vi "HFRR ADV v024 new software.vi"() -> ()   [LabVIEW 2025] (continued)
                  n3489 = property on="Air Temperature  ( °C )" class="XYGraph (strict)"("Y Scale.Name Label.Text"=w4683) -> ()  [unwired: 2 in, 2 out]
                }
                frame 82 {
                  n3490 = local write "S 84"(w4684) -> ()
                }
                frame 83 {
                  n3491 = local write "S 85"(w4685) -> ()
                }
                frame 84 {
                  n3492 = local write "S 86"(w4686) -> ()
                }
                frame 85 {
                  n3493 = local write "S 87"(w4687) -> ()
                }
                frame 86 {
                  n3494 = local write "S 88"(w4688) -> ()
                }
                frame 87 {
                }
                frame 88 {
                  n3495 = local write "S 90"(w4690) -> ()
                }
                frame 89 {
                  n3496 = local write "S 91"(w4691) -> ()
                }
                frame 90 {
                  n3497 = local write "S 92"(w4692) -> ()
                }
                frame 91 {
                  n3498 = local write "S 93"(w4693) -> ()
                }
                frame 92 {
                  n3499 = local write "S 94"(w4694) -> ()
                }
                frame 93 {
                  n3500 = local write "S 95"(w4695) -> ()
                }
                frame 94 {
                  n3501 = local write "S 96"(w4696) -> ()
                }
                frame 95 {
                  n3502 = local write "S 97"(w4697) -> ()
                }
                frame 96 {
                  n3503 = local write "S 98"(w4698) -> ()
                }
                frame 97 {
                  n3504 = local write "S 99"(w4699) -> ()
                }
                frame 98 {
                  n3505 = local write "S 100"(w4700) -> ()
                }
                frame 99 {
                  n3506 = local write "S 101"(w4701) -> ()
                }
                frame 100 {
                  n3507 = local write "S 102"(w4702) -> ()
                }
                frame 101 {
                  n3508 = local write "S 103"(w4703) -> ()
                }
                frame 102 {
                  n3509 = local write "S 104"(w4704) -> ()
                }
                frame 103 {
                  n3510 = local write "S 105"(w4705) -> ()
                }
                frame 104 {
                  n3511 = local write "S 106"(w4706) -> ()
                }
                frame 105 {
                }
                frame 106 {
                  n3512 = property on="OK Button 17" class="Bool (strict)"("Boolean Text.Text"=w4707) -> ()  [unwired: 2 in, 2 out]
                }
                frame 107 {
                  n3513 = property on="OK Button 16" class="Bool (strict)"("Boolean Text.Text"=w4708) -> ()  [unwired: 2 in, 2 out]
                }
                frame 108 {
                  n3514 = property on="TITTLE" class="Str"("Caption.Text"=w4709) -> ()  [unwired: 2 in, 2 out]
                }
                frame 109 {
                  "String 30" <- w4710
                }
                frame 110 {
                  n3515 = property on="Test Date" class="Str"("Caption.Text"=w4711) -> ()  [unwired: 2 in, 2 out]
                  "String 31" <- w4711
                }
                frame 111 {
                  n3516 = property on="Sample ID" class="Str"("Caption.Text"=w4712) -> ()  [unwired: 2 in, 2 out]
                  "String 32" <- w4712
                }
                frame 112 {
                  n3517 = property on="Tested by" class="Str"("Caption.Text"=w4713) -> ()  [unwired: 2 in, 2 out]
                  "String 33" <- w4713
                }
                frame 113 {
                  n3518 = property on="System Configured Printers 2" class="Arr (strict)"("Caption.Text"=w4714) -> ()  [unwired: 2 in, 2 out]
                }
                frame 114 {
                  n3519 = property on="Selected Printer" class="Str"("Caption.Text"=w4715) -> ()  [unwired: 2 in, 2 out]
                }
                frame 115 {
                  n3520 = property on="Select Printer 3" class="DigNum (strict)"("Caption.Text"=w4716) -> ()  [unwired: 2 in, 2 out]
                }
                frame 116 {
                  n3521 = property on="Print" class="Bool (strict)"("Boolean Text.Text"=w4717) -> ()  [unwired: 2 in, 2 out]
                }
                frame 117 {
                  "String 41" <- w4718
                }
                frame 118 {
                  n3522 = property on="tested by" class="Str"("Caption.Text"=w4719) -> ()  [unwired: 2 in, 2 out]
                }
                frame 119 {
                }
                frame 120 {
                  n3523 = property on="Export" class="Bool (strict)"("Boolean Text.Text"=w4720) -> ()  [unwired: 2 in, 2 out]
                }
                frame 121 {
                  n3524 = property on="TEMP INTERCEPT:" class="DigNum (strict)"("Caption.Text"=w4721) -> ()  [unwired: 2 in, 2 out]
                }
                frame 122 {
                  n3525 = property on="AIR TEMP INTERCEPT:" class="DigNum (strict)"("Caption.Text"=w4722) -> ()  [unwired: 2 in, 2 out]
                }
                frame 123 {
                  n3526 = property on="Select File Type" class="Enum (strict)"("Caption.Text"=w4723) -> ()  [unwired: 2 in, 2 out]
                }
                frame 124 {
                  n3527 = property on="s.NO" class="Str"("Caption.Text"=w4724) -> ()  [unwired: 2 in, 2 out]
                  "String 45" <- w4724
                }
                frame 125 {
                  n3528 = property on="trip1 8" class="Bool (strict)"("Boolean Text.Text"=w4725) -> ()  [unwired: 2 in, 2 out]
                }
                frame 126, Default {
                }
              }
            }
          }
          frame #1 {
            w4733 = TRUE ("Visible")
            n3529 = local read "S 91"() -> (w4750:string)
            n3530 = local read "S 90"() -> (w4749:string)
            n3531 = local read "S 88"() -> (w4748:string)
            n3532 = property on="File Path" class="Path"("Caption.Text"=w4749) -> ()  [unwired: 2 in, 2 out]
            n3533 = property on="SrvM CP" class="Bool (strict)"("Boolean Text.Text"=w4748) -> ()  [unwired: 2 in, 2 out]
            n3534 = local read "S 71"() -> (w4743:string)
            n3535 = local read "S 86"() -> (w4745:string)
            n3536 = local read "S 85"() -> (w4746:string)
            n3537 = local read "S 87"() -> (w4744:string)
            n3538 = local read "S 84"() -> (w4747:string)
            n3539 = local read "S 103"() -> (w4732:string)
            n3540 = local read "S 104"() -> (w4731:string)
            n3541 = property on="ENTER THE NEW PASSWORD" class="Str"("Caption.Text"=w4744) -> ()  [unwired: 2 in, 2 out]
            n3542 = property on="Password" class="Str"("Caption.Text"=w4746) -> ()  [unwired: 2 in, 2 out]
            n3543 = property on="ENTER CURRENT PASSWORD" class="Str"("Caption.Text"=w4745) -> ()  [unwired: 2 in, 2 out]
            n3544 = property on="EDIT" class="Bool (strict)"("Boolean Text.Text"=w4743) -> ()  [unwired: 2 in, 2 out]
            n3545 = property on="SAVE" class="Bool (strict)"("Boolean Text.Text"=w4747) -> ()  [unwired: 2 in, 2 out]
            n3546 = Build Array(w4732, w4731) -> (w4730:string[])
            n3547 = property on="Heater Button" class="Bool (strict)"("Strings [4]"=w4730) -> ()  [unwired: 2 in, 2 out]
            n3548 = local read "S 92"() -> (w4742:string)
            n3549 = local read "S 93"() -> (w4741:string)
            n3550 = local read "S 105"() -> (w4728:string)
            n3551 = local read "S 106"() -> (w4727:string)
            n3552 = Build Array(w4742, w4741) -> ()  [unwired: 1 out]
            n3553 = Build Array(w4728, w4727) -> (w4729:string[])
            n3554 = local read "S 95"() -> (w4739:string)
            n3555 = local read "S 94"() -> (w4740:string)
            n3556 = local read "bs"() -> (w4755:string)
            n3557 = local read "as"() -> (w4756:string)
            n3558 = property on="Humidity" class="Bool (strict)"("Strings [4]"=w4729) -> ()  [unwired: 2 in, 2 out]
            n3559 = Concatenate Strings(w4755, "\r", w4756) -> ()  [unwired: 1 out]
            n3560 = property on="STROKE GAIN :" class="DigNum (strict)"("Caption.Text"=w4739) -> ()  [unwired: 2 in, 2 out]
            n3561 = property on="DISPLACEMENT :" class="DigNum (strict)"("Caption.Text"=w4740) -> ()  [unwired: 2 in, 2 out]
            n3562 = property on="Rh After" class="DigNum (strict)"("Caption.Size to Text?"=TRUE ("Caption.Size to Text")) -> ()  [unwired: 2 in, 2 out]
            n3563 = local read "S 48"() -> (w4779:string)
            n3564 = local read "S 50"() -> (w4777:string)
            n3565 = local read "S 51"() -> (w4776:string)
            n3566 = local read "S 49"() -> (w4778:string)
            n3567 = local read "S 52"() -> (w4775:string)
            n3568 = local read "as"() -> (w4760:string)
            n3569 = local read "bs"() -> (w4761:string)
            n3570 = local read "S 56"() -> (w4774:string)
            n3571 = local read "S 57"() -> (w4773:string)
            n3572 = local read "S 58"() -> (w4772:string)
            n3573 = local read "S 59"() -> (w4771:string)
            n3574 = property on="OPEN" class="Bool (strict)"("Boolean Text.Text"=w4775) -> ()  [unwired: 2 in, 2 out]
            n3575 = property on="OPEN 1" class="Bool (strict)"("Boolean Text.Text"=w4779) -> ()  [unwired: 2 in, 2 out]
            n3576 = property on="OPEN 2" class="Bool (strict)"("Boolean Text.Text"=w4778) -> ()  [unwired: 2 in, 2 out]
            n3577 = property on="OPEN 3" class="Bool (strict)"("Boolean Text.Text"=w4777) -> ()  [unwired: 2 in, 2 out]
            n3578 = property on="OPEN 4" class="Bool (strict)"("Boolean Text.Text"=w4776) -> ()  [unwired: 2 in, 2 out]
            n3579 = Concatenate Strings(w4761, "\r", w4760) -> ()  [unwired: 1 out]
            n3580 = local read "S 102"() -> (w4734:string)
            n3581 = property on="КОФ1" class="DigNum (strict)"("Caption.Text"=w4774) -> ()  [unwired: 2 in, 2 out]
            n3582 = local read "S 98"() -> (w4738:string)
            n3583 = local read "S 99"() -> (w4737:string)
            n3584 = local read "S 100"() -> (w4736:string)
            n3585 = local read "S 101"() -> (w4735:string)
            n3586 = property on="КОФ2" class="DigNum (strict)"("Caption.Text"=w4773) -> ()  [unwired: 2 in, 2 out]
            n3587 = property on="КОФ3" class="DigNum (strict)"("Caption.Text"=w4772) -> ()  [unwired: 2 in, 2 out]
            n3588 = property on="КОФ4" class="DigNum (strict)"("Caption.Text"=w4771) -> ()  [unwired: 2 in, 2 out]
            n3589 = local read "bs"() -> (w4759:string)
            n3590 = local read "as"() -> (w4758:string)
            n3591 = local read "S 60"() -> (w4770:string)
            n3592 = local read "S 54"() -> (w4780:string)
            n3593 = Concatenate Strings(w4759, "\r", w4758) -> ()  [unwired: 1 out]
            n3594 = Concatenate Strings(w4780, w4770) -> ()  [unwired: 1 out]
            n3595 = local read "S 77"() -> (→"String 43":string)
            n3596 = local read "S 76"() -> (w4753:string)
            n3597 = local read "S 78"() -> (w4752:string)
            n3598 = local read "S 71"() -> (w4764:string)
            n3599 = local read "S 66"() -> (w4769:string)
            n3600 = local read "S 67"() -> (w4768:string)
            n3601 = local read "S 68"() -> (w4767:string)
            n3602 = local read "S 69"() -> (w4766:string)
            n3603 = local read "S 70"() -> (w4765:string)
            n3604 = property on="AIR TEMP" class="DigNum (strict)"("Caption.Text"=w4752) -> ()  [unwired: 2 in, 2 out]
            n3605 = property on="Set Strk" class="DigNum (strict)"("Caption.Text"=w4753) -> ()  [unwired: 2 in, 2 out]
            n3606 = property on="FRIC. FORCE :" class="DigNum (strict)"("Caption.Text"=w4769) -> ()  [unwired: 2 in, 2 out]
            n3607 = property on="TEMPERATURE :" class="DigNum (strict)"("Caption.Text"=w4768) -> ()  [unwired: 2 in, 2 out]
            n3608 = property on="SPEED OUT:" class="DigNum (strict)"("Caption.Text"=w4767) -> ()  [unwired: 2 in, 2 out]
            n3609 = property on="AIR TEMPERATURE :" class="DigNum (strict)"("Caption.Text"=w4766) -> ()  [unwired: 2 in, 2 out]
            n3610 = property on="HUMIDITY:" class="DigNum (strict)"("Caption.Text"=w4765) -> ()  [unwired: 2 in, 2 out]
            n3611 = property on="EDIT" class="Bool (strict)"("Boolean Text.Text"=w4764) -> ()  [unwired: 2 in, 2 out]
            n3612 = local read "S 79"() -> (w4751:string)
          }
          frame #2 {
          }
        }
        n3613 = local write "Lan flag"(10.0 ("Lan flag")) -> ()
      }
      frame Enabled {
      }
    }
    n3614 = Wait (ms)(milliseconds to wait=u32 2000) -> ()  [unwired: 1 out]
    n3615 = local read "Quit"() -> (w4554:bool)
  }
  n3616 = while {
    shift-right: [w4786] -> _
    shift-left: _ -> [w4787]
    shift-right: [w4784] -> _
    shift-left: T18 {"Read Heave and Surge"="", "Bytes at Heave Port"=0.0, "Heave and Surge COM Port:"="COM9", "Com Port 2"="COM7", "Residual Due"="", "Heave COM Status 2"=TRUE, "Heave COM Status"=TRUE, "Port 2"=TRUE, "Sway PPR"=6400.0, "Surge PPR"=6400.0, "Heave PPR"=6400.0, "Sway Pitch"=2.0, "Surge Pitch"=3.0, "Heave Pitch"=4.0, "Sway Pulses/mm"=320.0, "Surge Pulses/mm"=1600.0, "Heave Pulses/mm"=1600.0, "inner loop"=0.0, "Read Heave and Surge 2"="", "String 36"="", "Write S"=FALSE, "WriteCC1"=[""], "Heave COM Loop"=0, "LastCom"="", "EXIT"=FALSE, "Error Heave"={"status"=TRUE, "code"=-1073807343, "source"=""}} -> [w4783]
    shift-right: [w4781] -> _
    shift-left: enum16{"init", "MAIN", "Panel Close"}."init" -> [w4782]
    stop <- w4785 stop-if-true
    # "HUMIDITY LOOP LOGIC"
    n3617 = case shown="\"MAIN\"" w4782 {
      tunnel: w4787 -> [w4801 w4818 w4875 w4877]
      tunnel: [w4796 w4823 w4875 w4877] -> w4786
      tunnel: [_ _ TRUE _] -> w4785
      tunnel: [w4793 w4821 w4873 w4876] -> w4784
      tunnel: w4783 -> [w4798 w4817 w4873 w4876]
      tunnel: [enum16{"init", "MAIN", "Panel Close"}."MAIN" w4812 _ _] -> w4781
      frame "init" {
        n3618 = local read "Com Port 1"() -> (w4790:refnum<visa-resource-name>)
        n3619 = Bundle By Name(cluster=w4798, "Heave and Surge COM Port:"=w4790) -> (w4797:T18)
        n3620 = call "Instrument fgv uno.vi"("Enum"=T31."INIT", "error in (no error) 2"=w4801, "INPUT"=w4797) -> ("error"=w4799:errorcluster, "output"=w4795:T18)  [unwired: 6 in, 1 out]
        n3621 = case shown="Error" w4799 {
          selector: w4799 -> [w4803 _]
          tunnel: [w4803 w4807] -> w4796
          tunnel: w4795 -> [w4802 w4805]
          tunnel: [w4802 w4804] -> w4794
          frame No Error {
          }
          frame Error {
            n3622 = call "Instrument fgv uno.vi"("Enum"=T31."ERROR INIT", "INPUT"=w4805) -> ("error"=w4808:errorcluster, "output"=w4804:T18)  [unwired: 7 in, 1 out]
            n3623 = call <vilib>:"Clear Errors.vi"("error in (no error)"=w4808) -> ("error out"=w4807:errorcluster)  [unwired: 5 in, 1 out]
          }
        }
        n3624 = local read "LastCom Humidity"() -> (w4789:string)
        n3625 = Unbundle By Name(w4794) -> ("Heave COM Status 2"=→"COM Status":bool, "Error Heave"=→"Error  2":errorcluster)  [unwired: 1 out]
        n3626 = Bundle By Name(cluster=w4794, "LastCom"=w4789) -> (w4793:T18)
      }
      frame "MAIN" {
        n3627 = Unbundle By Name(w4817) -> ("Com Port 2"=w4825:refnum<visa-resource-name>)
        n3628 = local read "Com Port 1"() -> (w4811:refnum<visa-resource-name>)
        n3629 = local write "Com Port 5"(w4825) -> ()
        n3630 = Bundle By Name(cluster=w4817, "Heave and Surge COM Port:"=w4811) -> (w4816:T18)
        n3631 = Equal?(x=w4825, y=w4811) -> (x = y?=w4824:bool)
        n3632 = case shown="True" w4824 {
          tunnel: [w4829 w4846] -> w4823
          tunnel: w4818 -> [w4830 w4852]
          tunnel: w4816 -> [w4828 w4850]
          tunnel: [w4827 w4845] -> w4821
          frame False {
            n3633 = call <vilib>:"Clear Errors.vi"("error in (no error)"=w4830) -> ("error out"=w4826:errorcluster)  [unwired: 5 in, 1 out]
            n3634 = call "Instrument fgv uno.vi"("Enum"=T31."ERROR INIT", "error in (no error) 2"=w4826, "INPUT"=w4828) -> ("error"=w4832:errorcluster, "output"=w4827:T18)  [unwired: 6 in, 1 out]
            n3635 = call <vilib>:"Clear Errors.vi"("error in (no error)"=w4832) -> ("error out"=w4829:errorcluster)  [unwired: 5 in, 1 out]
          }
          frame True {
            n3636 = call "Instrument fgv uno.vi"("Enum"=T31."READ", "error in (no error) 2"=w4852, "INPUT"=w4850) -> ("error"=w4851:errorcluster, "output"=w4843:T18)  [unwired: 6 in, 1 out]
            n3637 = Bundle By Name(cluster=w4843, "String 36"="WRITE HUMIDITY") -> (w4842:T18)
            n3638 = case shown="True" "Write" {
              selector: "Write" -> [_ w4872]
              tunnel: w4851 -> [w4865 w4871]
              tunnel: [w4865 w4870] -> w4840
              tunnel: w4842 -> [w4864 w4867]
              tunnel: [w4864 w4866] -> w4839
              frame False {
              }
              frame True {
                n3639 = Not(x=w4872) -> (.not. x?=w4868:bool)
                n3640 = local write "Write"(w4868) -> ()
                n3641 = call "Instrument fgv uno.vi"("Enum"=T31."MANUAL WRITE", "error in (no error) 2"=w4871, "INPUT"=w4867) -> ("error"=w4870:errorcluster, "output"=w4866:T18)  [unwired: 6 in, 1 out]
              }
            }
            n3642 = Array Size(array="WriteHumidity") -> (size(s)=w4837:i32)
            n3643 = Greater Than 0?(x=w4837) -> (x > 0?=w4836:bool)
            n3644 = call "Instrument fgv uno.vi"("Enum"=T31."WRITE", "error in (no error) 2"=w4840, "WriteCC1"="WriteHumidity", "INPUT"=w4839) -> ("error"=w4848:errorcluster, "WriteCC1 2"=w4838:string[], "output"=w4847:T18)  [unwired: 5 in]
            n3645 = case shown="True" w4836 {
              tunnel: w4838 -> [_ w4854]
              frame False {
              }
              frame True {
                n3646 = local write "WriteHumidity"(w4854) -> ()
              }
            }
            n3647 = case shown="No Error" w4848 {
              selector: w4848 -> [w4855 w4858]
              tunnel: w4847 -> [w4856 w4863]
              tunnel: [w4856 w4862] -> w4845
              tunnel: [w4855 w4860] -> w4846
              frame No Error {
              }
              frame Error {
                n3648 = call <vilib>:"Clear Errors.vi"("error in (no error)"=w4858) -> ("error out"=w4857:errorcluster)  [unwired: 5 in, 1 out]
                n3649 = call "Instrument fgv uno.vi"("Enum"=T31."ERROR INIT", "error in (no error) 2"=w4857, "INPUT"=w4863) -> ("error"=w4861:errorcluster, "output"=w4862:T18)  [unwired: 6 in, 1 out]
                n3650 = call <vilib>:"Clear Errors.vi"("error in (no error)"=w4861) -> ("error out"=w4860:errorcluster)  [unwired: 5 in, 1 out]
              }
            }
            n3651 = Unbundle By Name(w4845) -> ("LastCom"=→"LastCom Humidity":string, "Read Heave and Surge"=→"Read HUMIDITY":string)
          }
        }
        n3652 = Unbundle By Name(w4821) -> ("Heave COM Status 2"=w4822:bool, "Error Heave"=w4819:errorcluster, "Bytes at Heave Port"=→"Bytes at Humidity Port  2":dbl)  [unwired: 1 out]
        n3653 = Unbundle By Name(w4819) -> ("status"=→"Humidity Port":bool)
        n3654 = Not(x=w4822) -> (.not. x?=w4809:bool)
        n3655 = local read "Quit"() -> (w4813:bool)
        n3656 = local write "COM Status"(w4809) -> ()
        n3657 = Select(t=enum16{"init", "MAIN", "Panel Close"}."Panel Close", s=w4813, f=enum16{"init", "MAIN", "Panel Close"}."MAIN") -> (s? t:f=w4812:enum16{"init", "MAIN", "Panel Close"})
      }
      frame "Panel Close" {
      }
      frame Default {
      }
    }
  }
  n3658 = disable-structure shown="Disabled" {
    frame Disabled {
      n3659 = while {
        tunnel: [w4879] -> _
        i -> [w4879]
        stop <- w4878 continue-if-true
        n3660 = Wait (ms)(milliseconds to wait=u32 50) -> ()  [unwired: 1 out]
        n3661 = stacked-sequence {
          frame #0 {
            # "Controls Text color"
            # "Controls BG color"
            n3662 = property on="FILE" class="Str"("Text.Text Colors:Text Color"="SC  Text") -> ()  [unwired: 2 in, 2 out]
            n3663 = property on="Fuel Discription :" class="Str"("Text.Text Colors:Text Color"="SC  Text") -> ()  [unwired: 2 in, 2 out]
            n3664 = property on="tested by" class="Str"("Text.Text Colors:Text Color"="SC  Text") -> ()  [unwired: 2 in, 2 out]
            n3665 = property on="Remarks :" class="Str"("Text.Text Colors:Text Color"="SC  Text") -> ()  [unwired: 2 in, 2 out]
            n3666 = property class="DigNum (strict)"("Numeric Text.Text Colors:BG Color"="NC BG") -> ()  [unwired: 2 in, 2 out]
            n3667 = property class="DigNum (strict)"("Numeric Text.Text Colors:BG Color"="NC BG") -> ()  [unwired: 2 in, 2 out]
            n3668 = property class="DigNum (strict)"("Numeric Text.Text Colors:BG Color"="NC BG") -> ()  [unwired: 2 in, 2 out]
            n3669 = property class="DigNum (strict)"("Numeric Text.Text Colors:BG Color"="NC BG") -> ()  [unwired: 2 in, 2 out]
            n3670 = property class="DigNum (strict)"("Numeric Text.Text Colors:BG Color"="NC BG") -> ()  [unwired: 2 in, 2 out]
            n3671 = property class="DigNum (strict)"("Numeric Text.Text Colors:BG Color"="NC BG") -> ()  [unwired: 2 in, 2 out]
            n3672 = property class="DigNum (strict)"("Numeric Text.Text Colors:BG Color"="NC BG") -> ()  [unwired: 2 in, 2 out]
            n3673 = property class="DigNum (strict)"("Numeric Text.Text Colors:BG Color"="NC BG") -> ()  [unwired: 2 in, 2 out]
            n3674 = property class="DigNum (strict)"("Numeric Text.Text Colors:BG Color"="NC BG") -> ()  [unwired: 2 in, 2 out]
            n3675 = property class="DigNum (strict)"("Numeric Text.Text Colors:BG Color"="NC BG") -> ()  [unwired: 2 in, 2 out]
            n3676 = property class="DigNum (strict)"("Numeric Text.Text Colors:BG Color"="NC BG") -> ()  [unwired: 2 in, 2 out]
            n3677 = property class="DigNum (strict)"("Numeric Text.Text Colors:BG Color"="NC BG") -> ()  [unwired: 2 in, 2 out]
            n3678 = property on="FILE" class="Str"("Text.Text Colors:BG Color"="SC BG 3") -> ()  [unwired: 2 in, 2 out]
            n3679 = property on="Fuel Discription :" class="Str"("Text.Text Colors:BG Color"="SC BG 3") -> ()  [unwired: 2 in, 2 out]
            n3680 = property on="tested by" class="Str"("Text.Text Colors:BG Color"="SC BG 3") -> ()  [unwired: 2 in, 2 out]
            n3681 = property on="Remarks :" class="Str"("Text.Text Colors:BG Color"="SC BG 3") -> ()  [unwired: 2 in, 2 out]
            n3682 = property class="DigNum (strict)"("Numeric Text.Text Colors:Text Color"="NC Text") -> ()  [unwired: 2 in, 2 out]
            n3683 = property class="DigNum (strict)"("Numeric Text.Text Colors:Text Color"="NC Text") -> ()  [unwired: 2 in, 2 out]
            n3684 = property class="DigNum (strict)"("Numeric Text.Text Colors:Text Color"="NC Text") -> ()  [unwired: 2 in, 2 out]
            n3685 = property class="DigNum (strict)"("Numeric Text.Text Colors:Text Color"="NC Text") -> ()  [unwired: 2 in, 2 out]
            n3686 = property class="DigNum (strict)"("Numeric Text.Text Colors:Text Color"="NC Text") -> ()  [unwired: 2 in, 2 out]
            n3687 = property class="DigNum (strict)"("Numeric Text.Text Colors:Text Color"="NC Text") -> ()  [unwired: 2 in, 2 out]
            n3688 = property class="DigNum (strict)"("Numeric Text.Text Colors:Text Color"="NC Text") -> ()  [unwired: 2 in, 2 out]
            n3689 = property class="DigNum (strict)"("Numeric Text.Text Colors:Text Color"="NC Text") -> ()  [unwired: 2 in, 2 out]
            n3690 = property class="DigNum (strict)"("Numeric Text.Text Colors:Text Color"="NC Text") -> ()  [unwired: 2 in, 2 out]
            n3691 = property class="DigNum (strict)"("Numeric Text.Text Colors:Text Color"="NC Text") -> ()  [unwired: 2 in, 2 out]
            n3692 = property class="DigNum (strict)"("Numeric Text.Text Colors:Text Color"="NC Text") -> ()  [unwired: 2 in, 2 out]
            n3693 = property class="DigNum (strict)"("Numeric Text.Text Colors:Text Color"="NC Text") -> ()  [unwired: 2 in, 2 out]
            n3694 = property class="DigNum (strict)"("Numeric Text.Text Colors:Text Color"="NI Text  2") -> ()  [unwired: 2 in, 2 out]
            n3695 = property class="DigNum (strict)"("Numeric Text.Text Colors:Text Color"="NI Text  2") -> ()  [unwired: 2 in, 2 out]
            n3696 = property class="DigNum (strict)"("Numeric Text.Text Colors:Text Color"="NI Text  2") -> ()  [unwired: 2 in, 2 out]
            n3697 = property class="DigNum (strict)"("Numeric Text.Text Colors:Text Color"="NI Text  2") -> ()  [unwired: 2 in, 2 out]
            n3698 = property class="DigNum (strict)"("Numeric Text.Text Colors:Text Color"="NI Text  2") -> ()  [unwired: 2 in, 2 out]
            n3699 = property class="DigNum (strict)"("Numeric Text.Text Colors:Text Color"="NI Text  2") -> ()  [unwired: 2 in, 2 out]
            n3700 = property class="DigNum (strict)"("Numeric Text.Text Colors:Text Color"="NI Text  2") -> ()  [unwired: 2 in, 2 out]
            n3701 = property class="DigNum (strict)"("Numeric Text.Text Colors:Text Color"="NI Text  2") -> ()  [unwired: 2 in, 2 out]
            n3702 = property class="DigNum (strict)"("Numeric Text.Text Colors:Text Color"="NI Text  2") -> ()  [unwired: 2 in, 2 out]
            n3703 = property class="DigNum (strict)"("Numeric Text.Text Colors:Text Color"="NI Text  2") -> ()  [unwired: 2 in, 2 out]
            n3704 = property class="DigNum (strict)"("Numeric Text.Text Colors:Text Color"="NI Text  2") -> ()  [unwired: 2 in, 2 out]
            n3705 = property class="DigNum (strict)"("Numeric Text.Text Colors:Text Color"="NI Text  2") -> ()  [unwired: 2 in, 2 out]
            n3706 = property class="DigNum (strict)"("Numeric Text.Text Colors:Text Color"="NI Text  2") -> ()  [unwired: 2 in, 2 out]
            n3707 = property class="DigNum (strict)"("Numeric Text.Text Colors:Text Color"="NI Text  2") -> ()  [unwired: 2 in, 2 out]
            n3708 = property class="DigNum (strict)"("Numeric Text.Text Colors:Text Color"="NI Text  2") -> ()  [unwired: 2 in, 2 out]
            n3709 = property on="Coefficient Of Friction" class="XYGraph (strict)"("Plot Area:Colors:FG Color"="GFG  2", "Plot Area:Colors:BG Color"="GBG   2") -> ()  [unwired: 2 in, 2 out]
            n3710 = property on="Humidity ( %RH )" class="XYGraph (strict)"("Plot Area:Colors:FG Color"="GFG  2", "Plot Area:Colors:BG Color"="GBG   2") -> ()  [unwired: 2 in, 2 out]
            n3711 = property on="Air Temperature  ( °C )" class="XYGraph (strict)"("Plot Area:Colors:FG Color"="GFG  2", "Plot Area:Colors:BG Color"="GBG   2") -> ()  [unwired: 2 in, 2 out]
            n3712 = property on="Sample Temperature ( °C )" class="XYGraph (strict)"("Plot Area:Colors:FG Color"="GFG  2", "Plot Area:Colors:BG Color"="GBG   2") -> ()  [unwired: 2 in, 2 out]
            n3713 = property class="DigNum (strict)"("Numeric Text.Text Colors:BG Color"="NI BG 2") -> ()  [unwired: 2 in, 2 out]
            n3714 = property class="DigNum (strict)"("Numeric Text.Text Colors:BG Color"="NI BG 2") -> ()  [unwired: 2 in, 2 out]
            n3715 = property class="DigNum (strict)"("Numeric Text.Text Colors:BG Color"="NI BG 2") -> ()  [unwired: 2 in, 2 out]
            n3716 = property class="DigNum (strict)"("Numeric Text.Text Colors:BG Color"="NI BG 2") -> ()  [unwired: 2 in, 2 out]
            n3717 = property class="DigNum (strict)"("Numeric Text.Text Colors:BG Color"="NI BG 2") -> ()  [unwired: 2 in, 2 out]
            n3718 = property class="DigNum (strict)"("Numeric Text.Text Colors:BG Color"="NI BG 2") -> ()  [unwired: 2 in, 2 out]
            n3719 = property class="DigNum (strict)"("Numeric Text.Text Colors:BG Color"="NI BG 2") -> ()  [unwired: 2 in, 2 out]
            n3720 = property class="DigNum (strict)"("Numeric Text.Text Colors:BG Color"="NI BG 2") -> ()  [unwired: 2 in, 2 out]
            n3721 = property class="DigNum (strict)"("Numeric Text.Text Colors:BG Color"="NI BG 2") -> ()  [unwired: 2 in, 2 out]
            n3722 = property class="DigNum (strict)"("Numeric Text.Text Colors:BG Color"="NI BG 2") -> ()  [unwired: 2 in, 2 out]
            n3723 = property class="DigNum (strict)"("Numeric Text.Text Colors:BG Color"="NI BG 2") -> ()  [unwired: 2 in, 2 out]
            n3724 = property class="DigNum (strict)"("Numeric Text.Text Colors:BG Color"="NI BG 2") -> ()  [unwired: 2 in, 2 out]
            n3725 = property class="DigNum (strict)"("Numeric Text.Text Colors:BG Color"="NI BG 2") -> ()  [unwired: 2 in, 2 out]
            n3726 = property class="DigNum (strict)"("Numeric Text.Text Colors:BG Color"="NI BG 2") -> ()  [unwired: 2 in, 2 out]
            n3727 = property class="DigNum (strict)"("Numeric Text.Text Colors:BG Color"="NI BG 2") -> ()  [unwired: 2 in, 2 out]
            n3728 = property class="Bool"("Colors [4]"="Boolean BC T & BG") -> ()  [unwired: 2 in, 2 out]
            n3729 = property on="Save & Continue" class="Bool (strict)"("Colors [4]"="Boolean BC T & BG") -> ()  [unwired: 2 in, 2 out]
            n3730 = property on="Heater Button" class="Bool (strict)"("Colors [4]"="Boolean BC T & BG") -> ()  [unwired: 2 in, 2 out]
            n3731 = property class="Bool"("Colors [4]"="Boolean BC T & BG") -> ()  [unwired: 2 in, 2 out]
            n3732 = property on="Humidity" class="Bool (strict)"("Colors [4]"="Boolean BC T & BG") -> ()  [unwired: 2 in, 2 out]
            n3733 = property class="Bool (strict)"("Colors [4]"="Boolean BC T & BG") -> ()  [unwired: 2 in, 2 out]
            n3734 = property on="RUN" class="Bool (strict)"("Colors [4]"="Boolean BC T & BG") -> ()  [unwired: 2 in, 2 out]
            n3735 = property on="trip1 8" class="Bool (strict)"("Colors [4]"="Boolean BC T & BG") -> ()  [unwired: 2 in, 2 out]
            n3736 = property class="Bool"("Colors [4]"="Boolean BC T & BG") -> ()  [unwired: 2 in, 2 out]
            n3737 = property class="Bool (strict)"("Colors [4]"="Boolean BC T & BG") -> ()  [unwired: 2 in, 2 out]
            n3738 = property on="OPEN 1" class="Bool (strict)"("Colors [4]"="Boolean BC T & BG 2") -> ()  [unwired: 2 in, 2 out]
            n3739 = property on="OPEN 2" class="Bool (strict)"("Colors [4]"="Boolean BC T & BG 2") -> ()  [unwired: 2 in, 2 out]
            n3740 = property on="OPEN 3" class="Bool (strict)"("Colors [4]"="Boolean BC T & BG 2") -> ()  [unwired: 2 in, 2 out]
            n3741 = property on="OPEN 4" class="Bool (strict)"("Colors [4]"="Boolean BC T & BG 2") -> ()  [unwired: 2 in, 2 out]
            n3742 = property on="OPEN" class="Bool (strict)"("Colors [4]"="Boolean BC T & BG 2") -> ()  [unwired: 2 in, 2 out]
            n3743 = property on="rstv2" class="Bool"("Colors [4]"="Boolean BC T & BG 2") -> ()  [unwired: 2 in, 2 out]
            n3744 = property on="RST CP" class="Bool"("Colors [4]"="Boolean BC T & BG 2") -> ()  [unwired: 2 in, 2 out]
            n3745 = property on="RSTV1 3" class="Bool"("Colors [4]"="Boolean BC T & BG 2") -> ()  [unwired: 2 in, 2 out]
            n3746 = property on="RSTV1 2" class="Bool"("Colors [4]"="Boolean BC T & BG 2") -> ()  [unwired: 2 in, 2 out]
          }
          frame #1 {
          }
        }
        n3747 = local read "Quit"() -> (w4878:bool)
      }
    }
    frame Enabled {
    }
  }
  n3748 = while {
    shift-right: [w4896] -> _
    shift-left: _ -> [w4897]
    shift-right: [w4894] -> _
    shift-left: T18 {"Read Heave and Surge"="", "Bytes at Heave Port"=0.0, "Heave and Surge COM Port:"="COM9", "Com Port 2"="COM7", "Residual Due"="", "Heave COM Status 2"=TRUE, "Heave COM Status"=TRUE, "Port 2"=TRUE, "Sway PPR"=6400.0, "Surge PPR"=6400.0, "Heave PPR"=6400.0, "Sway Pitch"=2.0, "Surge Pitch"=3.0, "Heave Pitch"=4.0, "Sway Pulses/mm"=320.0, "Surge Pulses/mm"=1600.0, "Heave Pulses/mm"=1600.0, "inner loop"=0.0, "Read Heave and Surge 2"="", "String 36"="", "Write S"=FALSE, "WriteCC1"=[""], "Heave COM Loop"=0, "LastCom"="", "EXIT"=FALSE, "Error Heave"={"status"=TRUE, "code"=-1073807343, "source"=""}} -> [w4893]
    shift-right: [w4891] -> _
    shift-left: enum16{"init", "MAIN", "Panel Close"}."init" -> [w4892]
    stop <- w4895 stop-if-true
    # "UNO CODE LOGIC"
    n3749 = case shown="\"MAIN\"" w4892 {
      tunnel: w4897 -> [w4911 w4928 w4986 w4988]
      tunnel: [w4905 w4934 w4986 w4988] -> w4896
      tunnel: [_ _ TRUE _] -> w4895
      tunnel: [w4901 w4932 w4984 w4987] -> w4894
      tunnel: w4893 -> [w4908 w4927 w4984 w4987]
      tunnel: [enum16{"init", "MAIN", "Panel Close"}."MAIN" w4921 _ _] -> w4891
      frame "init" {
        n3750 = Bundle By Name(cluster=w4908, "Heave and Surge COM Port:"="C3 :") -> (w4907:T18)
        n3751 = call "Instrument fgv.vi"("Enum"=T31."INIT", "error in (no error) 2"=w4911, "INPUT"=w4907) -> ("error"=w4909:errorcluster, "output"=w4904:T18)  [unwired: 6 in, 1 out]
        n3752 = case shown="Error" w4909 {
          selector: w4909 -> [w4913 _]
          tunnel: [w4913 w4917] -> w4905
          tunnel: w4904 -> [w4912 w4915]
          tunnel: [w4912 w4914] -> w4902
          frame No Error {
          }
          frame Error {
            n3753 = call "Instrument fgv.vi"("Enum"=T31."ERROR INIT", "INPUT"=w4915) -> ("error"=w4918:errorcluster, "output"=w4914:T18)  [unwired: 7 in, 1 out]
            n3754 = call <vilib>:"Clear Errors.vi"("error in (no error)"=w4918) -> ("error out"=w4917:errorcluster)  [unwired: 5 in, 1 out]
          }
        }
        n3755 = local read "LastCom UNO"() -> (w4898:string)
        n3756 = Unbundle By Name(w4902) -> ("Heave COM Status 2"=→"Instrument Status":bool, "Error Heave"=→"Error":errorcluster)  [unwired: 1 out]
        n3757 = Bundle By Name(cluster=w4902, "LastCom"=w4898) -> (w4901:T18)
      }
      frame "MAIN" {
        n3758 = Unbundle By Name(w4927) -> ("Com Port 2"=w4936:refnum<visa-resource-name>)
        n3759 = local write "Com Port 4"(w4936) -> ()
        n3760 = local read "C3 :"() -> (w4925:refnum<visa-resource-name>)
        n3761 = Bundle By Name(cluster=w4927, "Heave and Surge COM Port:"=w4925) -> (w4926:T18)
        n3762 = Equal?(x=w4936, y=w4925) -> (x = y?=w4935:bool)
        n3763 = case shown="True" w4935 {
          tunnel: [w4940 w4957] -> w4934
          tunnel: w4928 -> [w4941 w4963]
          tunnel: w4926 -> [w4939 w4961]
          tunnel: [w4938 w4956] -> w4932
          frame False {
            n3764 = call <vilib>:"Clear Errors.vi"("error in (no error)"=w4941) -> ("error out"=w4937:errorcluster)  [unwired: 5 in, 1 out]
            n3765 = call "Instrument fgv.vi"("Enum"=T31."ERROR INIT", "error in (no error) 2"=w4937, "INPUT"=w4939) -> ("error"=w4943:errorcluster, "output"=w4938:T18)  [unwired: 6 in, 1 out]
            n3766 = call <vilib>:"Clear Errors.vi"("error in (no error)"=w4943) -> ("error out"=w4940:errorcluster)  [unwired: 5 in, 1 out]
          }
          frame True {
            n3767 = call "Instrument fgv.vi"("Enum"=T31."READ", "error in (no error) 2"=w4963, "INPUT"=w4961) -> ("error"=w4962:errorcluster, "output"=w4954:T18)  [unwired: 6 in, 1 out]
            n3768 = Bundle By Name(cluster=w4954, "String 36"="WRITE UNO") -> (w4953:T18)
            n3769 = case shown="True" "Write S" {
              selector: "Write S" -> [_ w4983]
              tunnel: w4962 -> [w4976 w4982]
              tunnel: [w4976 w4981] -> w4951
              tunnel: w4953 -> [w4975 w4978]
              tunnel: [w4975 w4977] -> w4950
              frame False {
              }
              frame True {
                n3770 = Not(x=w4983) -> (.not. x?=w4979:bool)
                n3771 = local write "Write S"(w4979) -> ()
                n3772 = call "Instrument fgv.vi"("Enum"=T31."MANUAL WRITE", "error in (no error) 2"=w4982, "INPUT"=w4978) -> ("error"=w4981:errorcluster, "output"=w4977:T18)  [unwired: 6 in, 1 out]
              }
            }
            n3773 = Array Size(array="Write UNO") -> (size(s)=w4948:i32)
            n3774 = Greater Than 0?(x=w4948) -> (x > 0?=w4947:bool)
            n3775 = call "Instrument fgv.vi"("Enum"=T31."WRITE", "error in (no error) 2"=w4951, "WriteCC1"="Write UNO", "INPUT"=w4950) -> ("error"=w4959:errorcluster, "WriteCC1 2"=w4949:string[], "output"=w4958:T18)  [unwired: 5 in]
            n3776 = case shown="True" w4947 {
              tunnel: w4949 -> [_ w4965]
              frame False {
              }
              frame True {
                n3777 = local write "Write UNO"(w4965) -> ()
              }
            }
            n3778 = case shown="Error" w4959 {
              selector: w4959 -> [w4966 w4969]
              tunnel: w4958 -> [w4967 w4974]
              tunnel: [w4967 w4973] -> w4956
              tunnel: [w4966 w4971] -> w4957
              frame No Error {
              }
              frame Error {
                n3779 = call <vilib>:"Clear Errors.vi"("error in (no error)"=w4969) -> ("error out"=w4968:errorcluster)  [unwired: 5 in, 1 out]
                n3780 = call "Instrument fgv.vi"("Enum"=T31."ERROR INIT", "error in (no error) 2"=w4968, "INPUT"=w4974) -> ("error"=w4972:errorcluster, "output"=w4973:T18)  [unwired: 6 in, 1 out]
                n3781 = call <vilib>:"Clear Errors.vi"("error in (no error)"=w4972) -> ("error out"=w4971:errorcluster)  [unwired: 5 in, 1 out]
              }
            }
            n3782 = Unbundle By Name(w4956) -> ("LastCom"=→"LastCom UNO":string, "Read Heave and Surge"=→"Read UNO":string)
          }
        }
        n3783 = Unbundle By Name(w4932) -> ("Heave COM Status 2"=w4933:bool, "Heave COM Status"=w4920:bool, "Error Heave"=w4930:errorcluster, "Bytes at Heave Port"=→"Bytes at Humidity Port":dbl)
        n3784 = Unbundle By Name(w4930) -> ()  [unwired: 1 out]
        n3785 = Not(x=w4920) -> (.not. x?=w4929:bool)
        n3786 = local write "Error"(w4930) -> ()
        n3787 = Not(x=w4933) -> (.not. x?=w4919:bool)
        n3788 = local write "Instrument Status"(w4929) -> ()
        n3789 = local write "Port 1a"(w4920) -> ()
        n3790 = local read "Quit"() -> (w4922:bool)
        n3791 = local write "COM Status"(w4919) -> ()
        n3792 = Select(t=enum16{"init", "MAIN", "Panel Close"}."Panel Close", s=w4922, f=enum16{"init", "MAIN", "Panel Close"}."MAIN") -> (s? t:f=w4921:enum16{"init", "MAIN", "Panel Close"})
      }
      frame "Panel Close" {
      }
      frame Default {
      }
    }
  }
  n3793 = while {
    stop <- w5014 stop-if-true
    n3794 = local read "Read HUMIDITY"() -> (w4989:string)
    n3795 = call <vilib>:"High Resolution Polling Wait.vi"("seconds to wait"=0.05) -> ()  [unwired: 10 in, 1 out]
    n3796 = Spreadsheet String To Array(delimiter (Tab)=",", format string="", spreadsheet string=w4989, array type (2D Dbl)=string[] []) -> (array=w5009:string[])
    n3797 = for {
      tunnel: w5009 -> [w5019] mode=indexing
      tunnel: string[] ["STATE;", "SET;", "RH;", "T;", "AMB_RH;", "AMB_T;", "PUMP;", "FAN_IN;", "FAN_OUT;", "DEHUM;", "CURRENT;", "STALL;"] -> [w5018] mode=indexing
      tunnel: [w5017] -> w5008 mode=indexing
      n3798 = Match Pattern(string=w5019, regular expression=w5018) -> (after substring=w5017:string)  [unwired: 1 in, 3 out]
    }
    n3799 = Index Array(array=w5008) -> (element #1=→"STATE :":string, element #2=→"SET :":string, element #3=w4997:string, element #4=→"T :":string, element #5=w4995:string, element #6=→"AMB_T :":string, element #7=→"PUMP :":string, element #8=→"FAN_IN :":string, element #9=→"FAN_OUT :":string, element #10=→"DEHUM :":string, element #11=→"CURRENT :":string, element #12=→"STALL :":string)  [unwired: 12 in]
    "RH :" <- w4997
    "AMB_RH :" <- w4995
    n3800 = Fract/Exp String To Number(string=w4997) -> (number=w4990:dbl)  [unwired: 3 in, 1 out]
    n3801 = Fract/Exp String To Number(string=w4995) -> (number=w4994:dbl)  [unwired: 3 in, 1 out]
    n3802 = local write "Ambient Humidity :"(w4994) -> ()
    n3803 = Equal?(x=w4990, y=0.0) -> (x = y?=w4992:bool)
    n3804 = case shown="True" w4992 {
      tunnel: [w5015 w5016] -> w4991
      tunnel: w4990 -> [w5015 _]
      frame False {
        (unwired) 0.0
        "Humidity temp" <- w5015
      }
      frame True {
        n3805 = local read "Humidity temp"() -> (w5016:dbl)
      }
    }
    "RH Numeric:" <- w4991
    n3806 = local read "Quit"() -> (w5014:bool)
  }
  n3807 = disable-structure shown="Disabled" {
    frame Disabled {
      n3808 = while {
        tunnel: [w5253] -> _
        i -> [w5253]
        stop <- w5250 stop-if-true
        n3809 = local read "powstat"() -> (w5251:bool)
        n3810 = case shown="True" w5251 {
          frame False {
          }
          frame True {
            n3811 = local read "RUN"() -> (w5254:bool)
            n3812 = case shown="True" w5254 {
              frame False {
                w5284 = 65.0 ("y")
                n3813 = local read "Set Hz"() -> (w5312:dbl)
                n3814 = local read "NORMAL LOAD"() -> (w5313:dbl)
                n3815 = Multiply(x=w5312, y=60.0) -> (x*y=w5319:dbl)
                n3816 = Multiply(x=1.2 ("y"), y=0.949) -> (x*y=w5288:dbl)
                n3817 = Multiply(x=1.2 ("y"), y=0.8166) -> (x*y=w5292:dbl)
                n3818 = Multiply(x=1.2 ("y"), y=0.851) -> (x*y=w5287:dbl)
                n3819 = local read "FF 2"() -> (w5311:dbl)
                n3820 = Absolute Value(x=w5319) -> (abs(x)=w5317:dbl)
                n3821 = case shown="13.." w5311 {
                  tunnel: [1 2 3] -> w5309
                  frame 0..10, Default {
                    # "Normal"
                  }
                  frame 11, 12 {
                  }
                  frame 13.. {
                  }
                }
                "FF STATE" <- w5309
                n3822 = local read "TEMP"() -> (w5272:dbl)
                n3823 = local read item#-1() -> (w5286)
                n3824 = Less?(x=w5286, y=w5292) -> (x < y?=w5289:bool)
                n3825 = In Range and Coerce(upper limit=w5288, x=w5286, lower limit=w5287) -> (In Range?=w5290:bool)  [unwired: 1 out]
                n3826 = case shown="3601.." w5317 {
                  tunnel: [1 2 3] -> w5315
                  frame 0..3000, Default {
                    # "Normal"
                  }
                  frame 3001..3600 {
                  }
                  frame 3601.. {
                  }
                }
                n3827 = case shown="11.." w5313 {
                  tunnel: [1 3] -> w5314
                  frame 1..10, Default {
                  }
                  frame 11.. {
                  }
                }
                "NL STATE" <- w5314
                n3828 = Multiply(x=1.2 ("y"), y=0.95) -> (x*y=w5302:dbl)
                n3829 = Multiply(x=w5284, y=0.954) -> (x*y=w5276:dbl)
                n3830 = Or(x=w5289, y=w5290) -> (x .or. y?=w5291:bool)
                n3831 = Greater Or Equal?(x=w5286, y=w5302) -> (x >= y?=w5299:bool)
                n3832 = Multiply(x=w5284, y=0.99) -> (x*y=w5273:dbl)
                n3833 = Greater Or Equal?(x=w5272, y=w5273) -> (x >= y?=w5278:bool)
                n3834 = Greater Or Equal?(x=w5272, y=w5276) -> (x >= y?=w5275:bool)
                n3835 = case shown="0, 1, Default" w5286 {
                  tunnel: [1 3] -> w5303
                  frame 0, 1, Default {
                  }
                  frame 2.. {
                  }
                }
                n3836 = case shown="True" w5299 {
                  tunnel: [1 3] -> w5304
                  frame False {
                  }
                  frame True {
                  }
                }
                n3837 = case shown="True" w5291 {
                  tunnel: [1 2] -> w5305
                  frame False {
                  }
                  frame True {
                  }
                }
                n3838 = case shown="..0" w5272 {
                  tunnel: [2 3 3 1] -> w5279
                  frame 61, 62 {
                  }
                  frame 63.. {
                  }
                  frame ..0 {
                  }
                  frame 10..60, Default {
                  }
                }
                n3839 = case shown="True" w5278 {
                  tunnel: [1 3] -> w5280
                  frame False {
                  }
                  frame True {
                  }
                }
                n3840 = Number To Decimal String(number=w5315) -> (decimal integer string=w5316:string)  [unwired: 1 in]
                n3841 = case shown="True" w5275 {
                  tunnel: [1 2] -> w5281
                  frame False {
                  }
                  frame True {
                  }
                }
                n3842 = Number To Decimal String(number=1) -> (decimal integer string=→"Air temp":string)  [unwired: 1 in]
                n3843 = Number To Decimal String(number=w5309) -> (decimal integer string=→"ff_st":string)  [unwired: 1 in]
                n3844 = local write "sp_st"(w5316) -> ()
                n3845 = Number To Decimal String(number=w5314) -> (decimal integer string=→"nl_st":string)  [unwired: 1 in]
                n3846 = Build Array(w5279, w5280, w5281) -> (w5282:i32[])
                n3847 = Build Array(w5303, w5304, w5305) -> (w5306:i32[])
                n3848 = Array Max & Min(array=w5282) -> (max value=w5283:i32)  [unwired: 3 out]
                n3849 = Array Max & Min(array=w5306) -> (max value=w5307:i32)  [unwired: 3 out]
                n3850 = Number To Decimal String(number=w5283) -> (decimal integer string=w5271:string)  [unwired: 1 in]
                n3851 = Number To Decimal String(number=w5307) -> (decimal integer string=→"Stroke Ln 2":string)  [unwired: 1 in]
                n3852 = local write "temp_st"(w5271) -> ()
              }
              frame True {
                w5369 = 65.0 ("y")
                # "Healthy -1\nWarning -2\nError -3"
                n3853 = local read "TEMP"() -> (w5380:dbl)
                n3854 = local read "NORMAL LOAD"() -> (w5384:dbl)
                n3855 = local read "Set Hz"() -> (w5382:dbl)
                n3856 = Multiply(x=1.2 ("y"), y=0.949) -> (x*y=w5364:dbl)
                n3857 = Multiply(x=1.2 ("y"), y=0.8166) -> (x*y=w5360:dbl)
                n3858 = Multiply(x=1.2 ("y"), y=0.851) -> (x*y=w5365:dbl)
                n3859 = Multiply(x=w5369, y=0.954) -> (x*y=w5376:dbl)
                n3860 = Multiply(x=w5369, y=0.99) -> (x*y=w5379:dbl)
                n3861 = Greater Or Equal?(x=w5380, y=w5379) -> (x >= y?=w5374:bool)
                n3862 = Multiply(x=w5382, y=60.0) -> (x*y=w5388:dbl)
                n3863 = Greater Or Equal?(x=w5380, y=w5376) -> (x >= y?=w5377:bool)
                n3864 = local read "FF 2"() -> (w5383:dbl)
                n3865 = local read item#-1() -> (w5366)
                n3866 = Less?(x=w5366, y=w5360) -> (x < y?=w5363:bool)
                n3867 = In Range and Coerce(upper limit=w5364, x=w5366, lower limit=w5365) -> (In Range?=w5362:bool)  [unwired: 1 out]
                n3868 = Absolute Value(x=w5388) -> (abs(x)=w5386:dbl)
                n3869 = case shown="63.." w5380 {
                  tunnel: [2 3 3 1] -> w5373
                  frame 61, 62 {
                  }
                  frame 63.. {
                  }
                  frame ..0 {
                  }
                  frame 10..60, Default {
                  }
                }
                n3870 = case shown="True" w5374 {
                  tunnel: [1 3] -> w5372
                  frame False {
                  }
                  frame True {
                  }
                }
                n3871 = case shown="True" w5377 {
                  tunnel: [1 2] -> w5371
                  frame False {
                  }
                  frame True {
                  }
                }
                n3872 = Multiply(x=1.2 ("y"), y=0.95) -> (x*y=w5350:dbl)
                n3873 = case shown="1..10, Default" w5384 {
                  tunnel: [1 3] -> w5391
                  frame 1..10, Default {
                  }
                  frame 11.. {
                  }
                }
                n3874 = case shown="0..10, Default" w5383 {
                  tunnel: [1 2 3] -> w5390
                  frame 0..10, Default {
                  }
                  frame 11, 12 {
                  }
                  frame 13.. {
                  }
                }
                n3875 = case shown="3601.." w5386 {
                  tunnel: [1 2 3] -> w5385
                  frame 0..3000, Default {
                    # "Normal"
                  }
                  frame 3001..3600 {
                  }
                  frame 3601.. {
                  }
                }
                n3876 = Or(x=w5363, y=w5362) -> (x .or. y?=w5361:bool)
                n3877 = Greater Or Equal?(x=w5366, y=w5350) -> (x >= y?=w5353:bool)
                n3878 = case shown="0, 1, Default" w5366 {
                  tunnel: [1 3] -> w5349
                  frame 0, 1, Default {
                  }
                  frame 2.. {
                  }
                }
                n3879 = case shown="True" w5353 {
                  tunnel: [1 3] -> w5348
                  frame False {
                  }
                  frame True {
                  }
                }
                n3880 = case shown="True" w5361 {
                  tunnel: [1 2] -> w5347
                  frame False {
                  }
                  frame True {
                  }
                }
                n3881 = Build Array(w5373, w5372, w5371) -> (w5370:i32[])
                n3882 = Number To Decimal String(number=w5385) -> (decimal integer string=→"sp_st":string)  [unwired: 1 in]
                n3883 = Array Max & Min(array=w5370) -> (max value=w5367:i32)  [unwired: 3 out]
                "TEMP STATE" <- w5367
                n3884 = Number To Decimal String(number=w5391) -> (decimal integer string=w5394:string)  [unwired: 1 in]
                n3885 = Number To Decimal String(number=w5390) -> (decimal integer string=w5392:string)  [unwired: 1 in]
                n3886 = Number To Decimal String(number=w5367) -> (decimal integer string=→"temp_st":string)  [unwired: 1 in]
                n3887 = Build Array(w5349, w5348, w5347) -> (w5346:i32[])
                n3888 = local write "nl_st"(w5394) -> ()
                n3889 = local write "ff_st"(w5392) -> ()
                n3890 = Number To Decimal String(number=1) -> (decimal integer string=w5389:string)  [unwired: 1 in]
                n3891 = Array Max & Min(array=w5346) -> (max value=w5345:i32)  [unwired: 3 out]
                n3892 = local write "Air temp"(w5389) -> ()
                n3893 = Number To Decimal String(number=w5345) -> (decimal integer string=w5344:string)  [unwired: 1 in]
                n3894 = local write "Stroke Ln 2"(w5344) -> ()
              }
            }
            n3895 = local read "Stroke Ln 2"() -> (w5256:string)
            n3896 = local read "nl_st"() -> (w5262:string)
            n3897 = local read "ff_st"() -> (w5259:string)
            n3898 = local read "sp_st"() -> (w5260:string)
            n3899 = local read "temp_st"() -> (w5261:string)
            n3900 = local read "Air temp"() -> (w5255:string)
            n3901 = Replace Array Subset(array="in", new element #1=w5262, index #1=1 ("index"), new element #2=w5259, index #2=2 ("index"), new element #3=w5261, index #3=3 ("index"), new element #4=w5260, index #4=4 ("index"), new element #5=w5256, index #5=5 ("index"), new element #6=w5255, index #6=6 ("index"), new element #7="Sensor State" ("new element/subarray"), index #7=0 ("index")) -> (→"out":string[])
          }
        }
        n3902 = Wait (ms)(milliseconds to wait=u32 10) -> ()  [unwired: 1 out]
        n3903 = local read "Quit"() -> (w5250:bool)
      }
      n3904 = while {
        stop <- w5225 stop-if-true
        n3905 = local read "run replace"() -> (w5227:bool)
        n3906 = Wait (ms)(milliseconds to wait=u32 100) -> ()  [unwired: 1 out]
        n3907 = Equal?(x="FLAG 2", y=0.0) -> (x = y?=w5228:bool)
        n3908 = case shown="True" w5228 {
          frame False {
          }
          frame True {
            n3909 = local write "FLAG 2"(100.0 ("FLAG 2")) -> ()
            n3910 = call <vilib>:"Read Characters From File.vi"("file path (dialog if empty)"=path "C:/LAB-IQ-NXT/WO 2449 TT.sig", "convert eol? (no:F)"=FALSE ("append to file? (new file:F)")) -> ("character string"=w5231:string)  [unwired: 4 in, 3 out]
            n3911 = call <vilib>:"Read Characters From File.vi"("file path (dialog if empty)"=path "C:/LAB-IQ-NXT/WO 2449 TRH.sig", "convert eol? (no:F)"=FALSE ("append to file? (new file:F)")) -> ("character string"=w5232:string)  [unwired: 4 in, 3 out]
            n3912 = Decimal String To Number(string=w5231) -> (number=w5233:i32)  [unwired: 2 in, 1 out]
            n3913 = local write "Total No. of Tests"(w5233) -> ()
            n3914 = Decimal String To Number(string=w5232) -> (number=w5236:i32)  [unwired: 2 in, 1 out]
            n3915 = local write "SEN.RUN HRS"(w5236) -> ()
          }
        }
        n3916 = case shown="True" w5227 {
          frame False {
          }
          frame True {
            n3917 = Equal?(x="FLAG 4", y=0.0) -> (x = y?=w5240:bool)
            n3918 = case shown="False" w5240 {
              frame False {
                n3919 = Get Date/Time In Seconds() -> (seconds since 1Jan1904=w5246:timestamp)
                n3920 = local read "START 3"() -> (w5244:dbl)
                n3921 = To Double Precision Float(number=w5246) -> (double precision float=w5245:dbl)
                n3922 = Subtract(x=w5245, y=w5244) -> (x-y=→"SENSOR TIME":dbl)
              }
              frame True {
                n3923 = Get Date/Time In Seconds() -> (seconds since 1Jan1904=w5248:timestamp)
                n3924 = local write "FLAG 4"(100.0 ("FLAG")) -> ()
                n3925 = To Double Precision Float(number=w5248) -> (double precision float=→"START 3":dbl)
              }
            }
          }
        }
        n3926 = local read "Quit"() -> (w5225:bool)
      }
      n3927 = while {
        shift-right: [w5025] -> _
        shift-left: _ -> [w5026]
        tunnel: [w5021] -> _
        i -> [w5021]
        stop <- w5020 stop-if-true
        n3928 = Wait (ms)(milliseconds to wait=u32 50 ("Refresh Rate (ms)")) -> ()  [unwired: 1 out]
        n3929 = local read "Json End Flg"() -> (w5022:bool)
        n3930 = Not(x="Upld AR 2") -> ()  [unwired: 1 out]
        n3931 = local read "Upld AR 2"() -> (w5023:bool)
        n3932 = call "Elapsed Time9"("Time Target (s)"="Sen.Upload Rate (s)", "Reset"=FALSE, "Auto Reset"=TRUE) -> ("Time has Elapsed"=w5032:bool)  [unwired: 9 in, 7 out]
        n3933 = Or(x=w5032, y=w5022) -> (x .or. y?=w5028:bool)
        n3934 = case shown="True" w5028 {
          frame False {
          }
          frame True {
            w5124 = "\"SensorName\":\"" ("string")
            w5094 = " \"},{"
            w5119 = "\",\"SensorState\":\""
            w5121 = "\",\"SensorModelNumber\":\"" ("string")
            w5120 = "\",\"SensorRuntimeHours\":\"" ("string")
            n3935 = local read "model num"() -> (w5118:string[])
            n3936 = local read "Sensor name"() -> (w5137:string[])
            n3937 = local read "run"() -> (w5108:string[])
            n3938 = local read "SENSOR TIME"() -> (w5064:dbl)
            n3939 = local read "out"() -> (w5057:string[])
            n3940 = local read "Total No. of Tests"() -> (w5062:dbl)
            n3941 = Select(t=60.0, s="Run test 3", f=3600.0) -> (s? t:f=w5072:dbl)
